vi "Read Measurement (Current and Voltage).vi"(6 "Wait Time (10 S)":i32=10, 7 "Voltage Buffer (smua.nvbuffer2)":string="smua.nvbuffer2", 8 "error in (no error)":errorcluster, 9 "Current Buffer (smua.nvbuffer1)":string="smua.nvbuffer1", 10 "Source Measure Unit Channel (0: Channel A)":i32(ring) items=["Channel A", "Channel B"], 11 "VISA resource name":refnum<visa-resource-name>) -> (0 "error out":errorcluster, 1 "Last Voltage (V)":dbl, 2 "Last Current (A)":dbl, 3 "VISA resource name out":refnum<visa-resource-name>, 4 "Voltage Buffer Data (V)":dbl[](array[numeric]), 5 "Current Buffer Data (A)":dbl[](array[numeric]))   [LabVIEW 2017, in "Keithley 2600 Series.lvlib"]
doc: "Returns the measured current and voltage."
uses:
  <instrlib>/Keithley 2600 Series/Keithley 2600 Series.lvlib
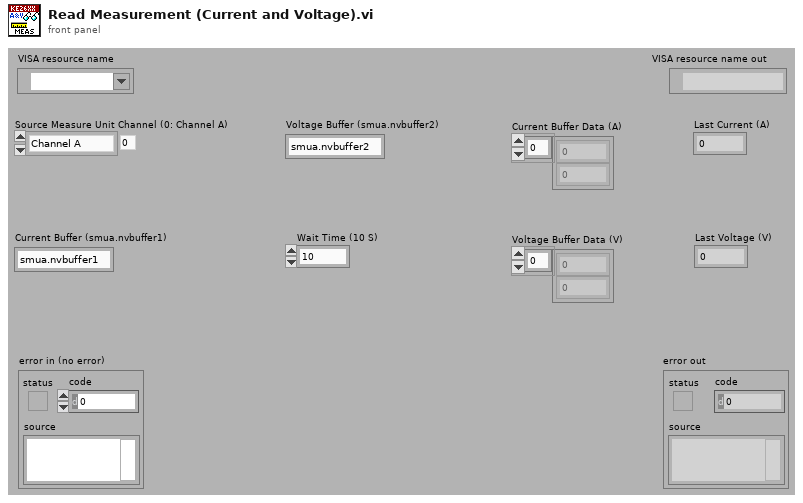
[diagram p1: front panel]
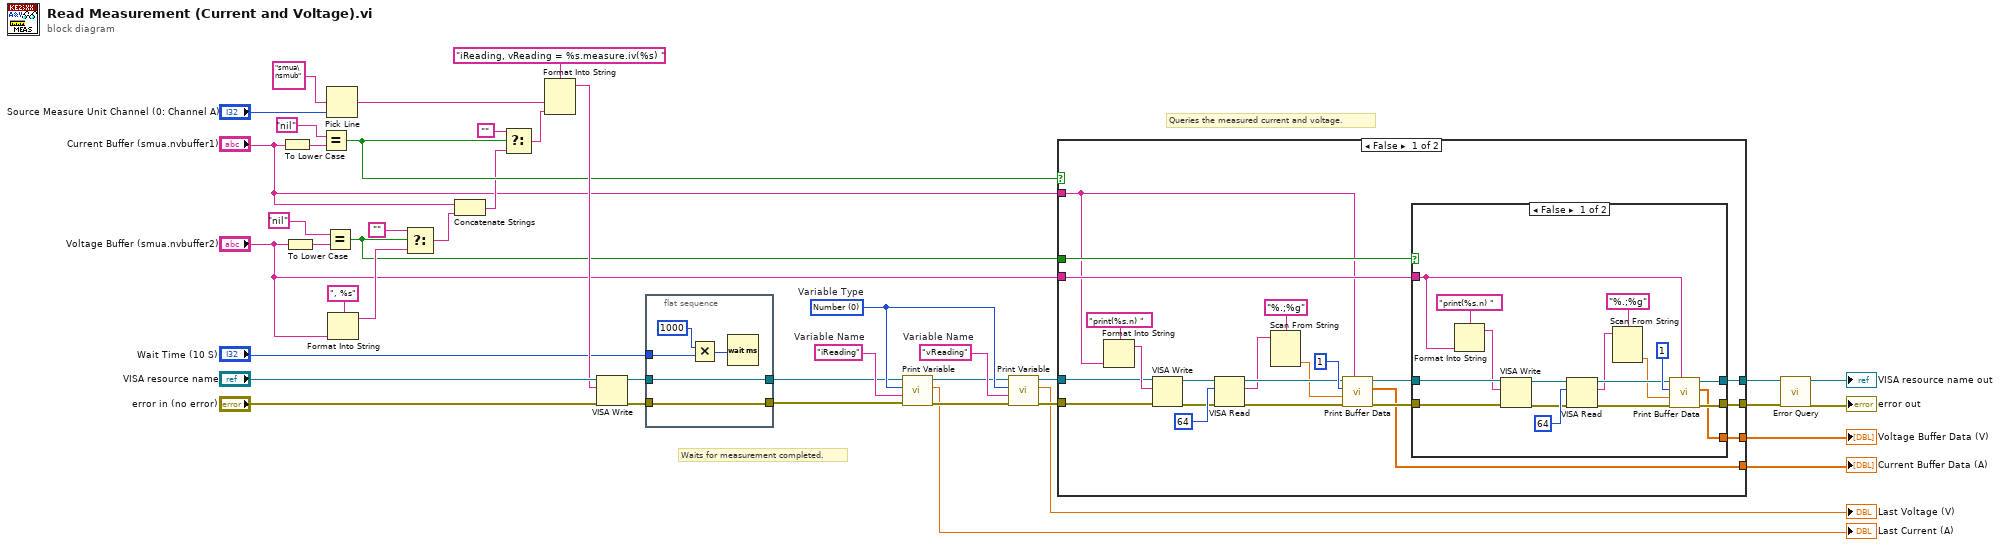
[diagram p0: block diagram]
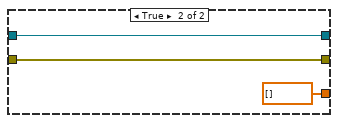
[diagram p2: hidden frame]
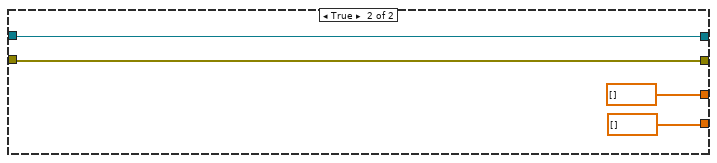
[diagram p3: hidden frame]
diagram:
  w10 = "vReading"  # Variable Name
  w11 = "iReading"  # Variable Name
  w9 = 0 items=["Number", "Message"]  # Variable Type
  # "Waits for measurement completed."
  # "Queries the measured current and voltage."
  n1 = To Lower Case(string="Current Buffer (smua.nvbuffer1)") -> (all lower case string=w14:string)
  n2 = To Lower Case(string="Voltage Buffer (smua.nvbuffer2)") -> (all lower case string=w15:string)
  n3 = Equal?(x="nil", y=w14) -> (x = y?=w26:bool)
  n4 = Equal?(x="nil", y=w15) -> (x = y?=w23:bool)
  n5 = Pick Line(multi-line string="smua\nsmub", line index="Source Measure Unit Channel (0: Channel A)") -> (output string=w35:string)  [unwired: 1 in]
  n6 = Format Into String(format string=", %s", "Voltage Buffer (smua.nvbuffer2)") -> (resulting string=w28:string)  [unwired: 2 in, 1 out]
  n7 = Select(t="", s=w23, f=w28) -> (s? t:f=w22:string)
  n8 = Concatenate Strings("Current Buffer (smua.nvbuffer1)", w22) -> (w21:string)
  n9 = Select(t="", s=w26, f=w21) -> (s? t:f=w32:string)
  n10 = Format Into String(format string="iReading, vReading = %s.measure.iv(%s) ", w35, w32) -> (resulting string=w27:string)  [unwired: 2 in, 1 out]
  n11 = VISA Write(VISA resource name="VISA resource name", write buffer=w27, error in (no error)="error in (no error)") -> (VISA resource name out=w18:refnum<visa-resource-name>, error out=w17:errorcluster)  [unwired: 1 out]
  n12 = flat-sequence {
    tunnel: [w47] -> w2
    tunnel: w18 -> [w47]
    tunnel: w17 -> [w43]
    tunnel: "Wait Time (10 S)" -> [w46]
    tunnel: [w43] -> w1
    frame #0 {
      n13 = Multiply(x=1000, y=w46) -> (x*y=w45:i32)
      n14 = Wait (ms)(milliseconds to wait=w45) -> ()  [unwired: 1 out]
    }
  }
  n15 = call <instrlib>:"Print Variable.vi"("error in (no error)"=w1, "Variable Name"=w11, "Variable Type (0: Number)"=w9, "VISA resource name"=w2) -> ("error out"=w7:errorcluster, "Number"=→"Last Current (A)":dbl, "VISA resource name out"=w8:refnum<visa-resource-name>)  [unwired: 4 in, 1 out]
  n16 = call <instrlib>:"Print Variable.vi"("error in (no error)"=w7, "Variable Name"=w10, "Variable Type (0: Number)"=w9, "VISA resource name"=w8) -> ("error out"=w5:errorcluster, "Number"=→"Last Voltage (V)":dbl, "VISA resource name out"=w6:refnum<visa-resource-name>)  [unwired: 4 in, 1 out]
  n17 = case shown="False" w26 {
    tunnel: [w54 w93] -> w25
    tunnel: w6 -> [w58 w93]
    tunnel: w5 -> [w57 w92]
    tunnel: [w53 w92] -> w24
    tunnel: w23 -> [w52 _]
    tunnel: "Current Buffer (smua.nvbuffer1)" -> [w50 _]
    tunnel: "Voltage Buffer (smua.nvbuffer2)" -> [w51 _]
    tunnel: [w49 dbl[] [] ("Buffer Data")] -> w20
    tunnel: [w48 dbl[] [] ("Buffer Data")] -> w19
    frame False {
      n18 = Format Into String(format string="print(%s.n) ", w50) -> (resulting string=w59:string)  [unwired: 2 in, 1 out]
      n19 = VISA Write(VISA resource name=w58, write buffer=w59, error in (no error)=w57) -> (VISA resource name out=w62:refnum<visa-resource-name>, error out=w61:errorcluster)  [unwired: 1 out]
      n20 = VISA Read(VISA resource name=w62, byte count=u32 64, error in (no error)=w61) -> (VISA resource name out=w67:refnum<visa-resource-name>, read buffer=w65:string, error out=w66:errorcluster)  [unwired: 1 out]
      n21 = Scan From String(format string="%.;%g", input string=w65) -> (output 1=w64:dbl)  [unwired: 3 in, 3 out]
      n22 = call <instrlib>:"Print Buffer Data.vi"("Reading Buffer (smua.nvbuffer1)"=w50, "error in (no error)"=w66, "End Index (1)"=w64, "Start Index (1)"=1 ("Start Index (0)"), "VISA resource name"=w67) -> ("error out"=w55:errorcluster, "Buffer Data"=w49:dbl[], "VISA resource name out"=w56:refnum<visa-resource-name>)  [unwired: 4 in]
      n23 = case shown="False" w52 {
        tunnel: w56 -> [w78 w89]
        tunnel: w55 -> [w77 w88]
        tunnel: [w76 w89] -> w54
        tunnel: [w75 w88] -> w53
        tunnel: w51 -> [w72 _]
        tunnel: [w71 dbl[] [] ("Buffer Data")] -> w48
        frame False {
          n24 = Format Into String(format string="print(%s.n) ", w72) -> (resulting string=w73:string)  [unwired: 2 in, 1 out]
          n25 = VISA Write(VISA resource name=w78, write buffer=w73, error in (no error)=w77) -> (VISA resource name out=w80:refnum<visa-resource-name>, error out=w79:errorcluster)  [unwired: 1 out]
          n26 = VISA Read(VISA resource name=w80, byte count=u32 64, error in (no error)=w79) -> (VISA resource name out=w84:refnum<visa-resource-name>, read buffer=w82:string, error out=w83:errorcluster)  [unwired: 1 out]
          n27 = Scan From String(format string="%.;%g", input string=w82) -> (output 1=w81:dbl)  [unwired: 3 in, 3 out]
          n28 = call <instrlib>:"Print Buffer Data.vi"("Reading Buffer (smua.nvbuffer1)"=w72, "error in (no error)"=w83, "End Index (1)"=w81, "Start Index (1)"=1 ("Start Index (0)"), "VISA resource name"=w84) -> ("error out"=w75:errorcluster, "Buffer Data"=w71:dbl[], "VISA resource name out"=w76:refnum<visa-resource-name>)  [unwired: 4 in]
        }
        frame True {
        }
      }
    }
    frame True {
    }
  }
  "Current Buffer Data (A)" <- w20
  "Voltage Buffer Data (V)" <- w19
  n29 = call <instrlib>:"Error Query.vi"("error in (no error)"=w24, "VISA resource name"=w25) -> ("error out"=→"error out":errorcluster, "VISA resource name out"=→"VISA resource name out":refnum<visa-resource-name>)  [unwired: 6 in, 2 out]
